vi "WriteCAlexFile.vi"(6 "Overwrite?(F)":bool, 8 "error in (no error)":errorcluster, 10 "Output Path":path, 11 "CAlexData":refnum<class "CAlexData2.lvclass">) -> (0 "error out":errorcluster, 1 "Actual File Name":string, 2 "Output Path dup":path, 3 "CAlexData 2":refnum<class "CAlexData2.lvclass">)   [LabVIEW 2015, in "CAlexData2.lvclass"]
uses:
  CAlexData2.lvclass
  CAlexData2.lvclass/CAlexData2.ctl
  ExpData/ExpData.lvclass
  CustomVIs/CustomVI.lvlib
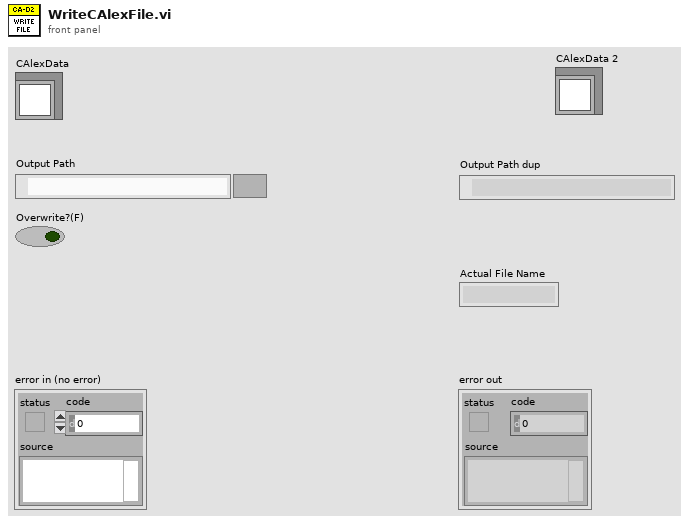
[diagram p1: front panel]
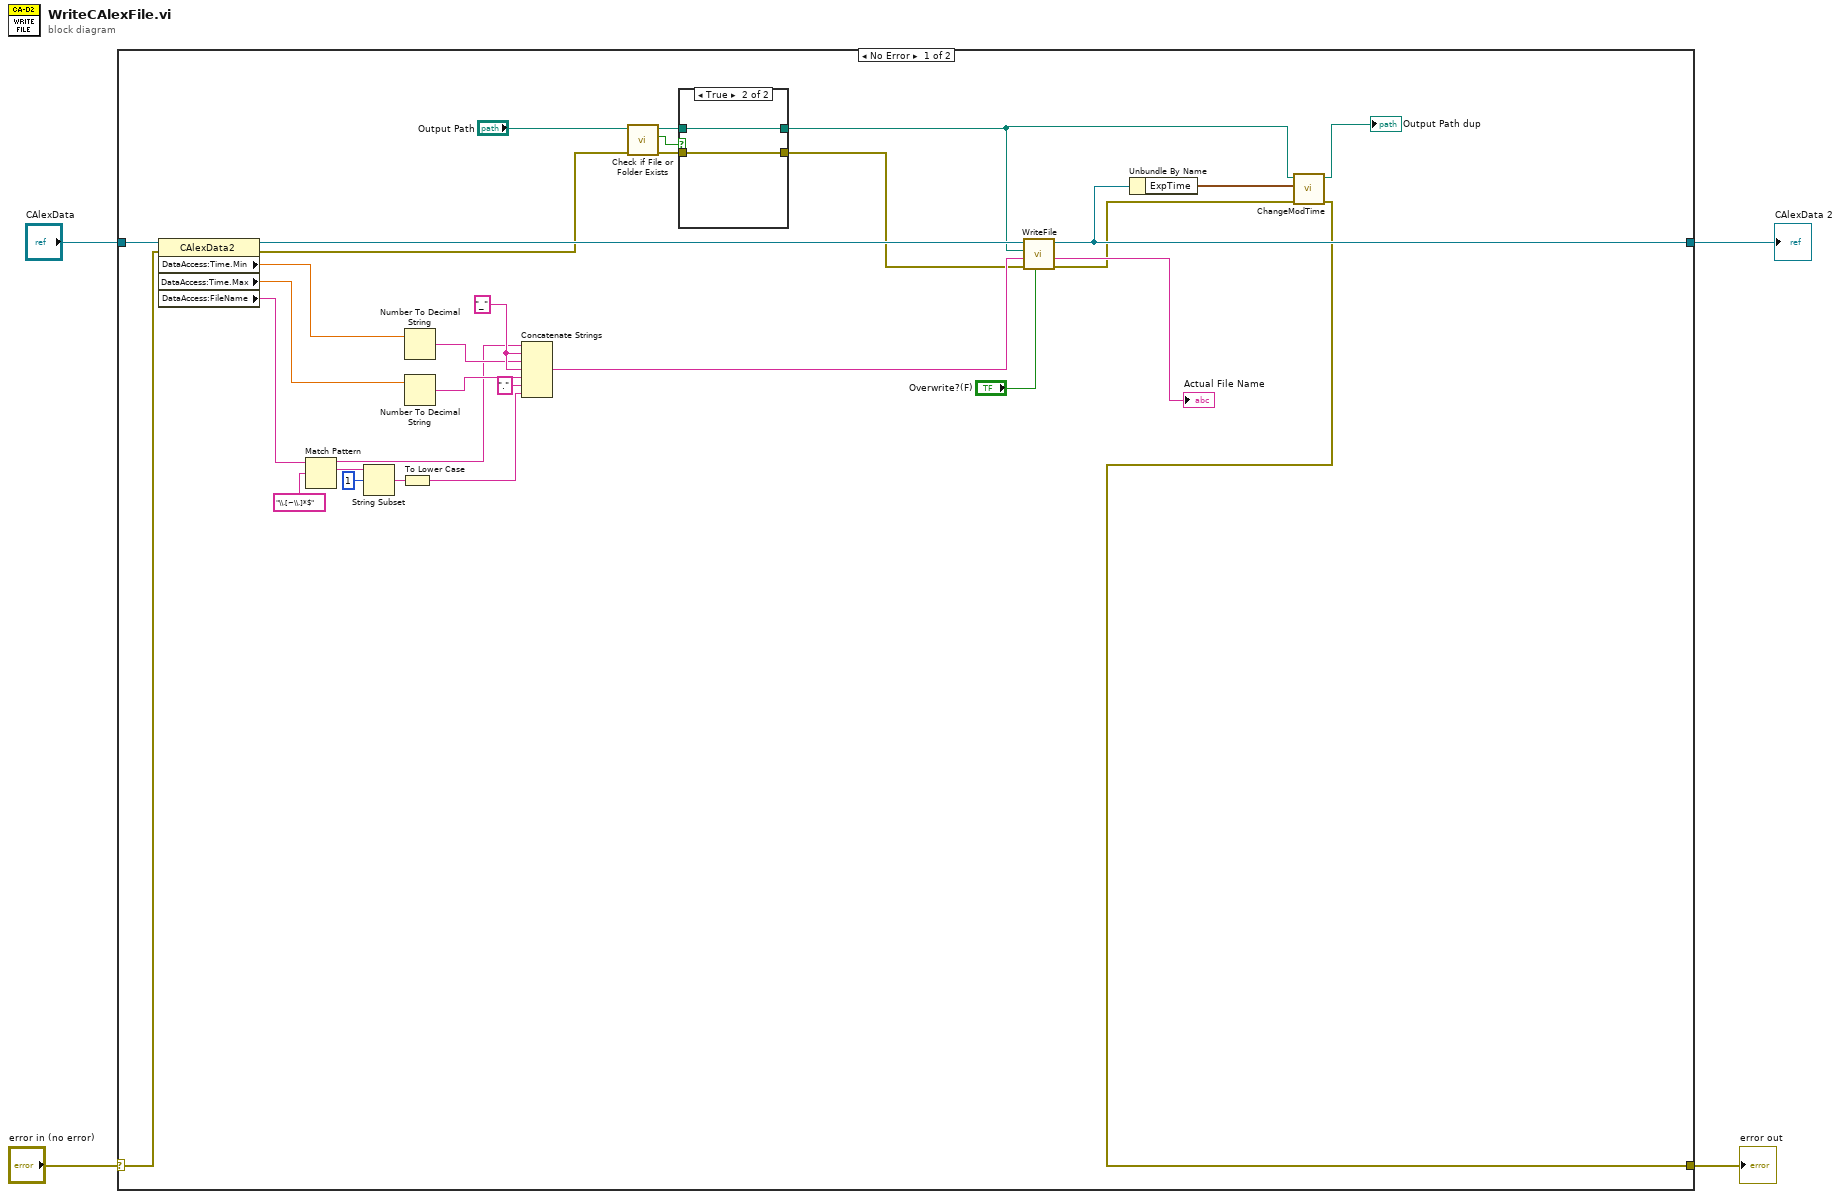
[diagram p0: block diagram]
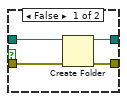
[diagram p2: hidden frame]
diagram:
  n1 = case shown="No Error" "error in (no error)" {
    selector: "error in (no error)" -> [w31 w43]
    tunnel: [w5 w43] -> w3
    tunnel: [w8 w42] -> w1
    tunnel: "CAlexData" -> [w33 w42]
    frame No Error {
      w28 = "_" ("string")
      n2 = property class="CAlexData2"(reference=w33, error in=w31) -> (reference out=w32:refnum<class "CAlexData2.lvclass">, error out=w20:errorcluster, "DataAccess:Time.Min"=w30:dbl, "DataAccess:Time.Max"=w29:dbl, "DataAccess:FileName"=w14:string)
      n3 = Match Pattern(string=w14, regular expression="\\.[~\\.]*$") -> (before substring=w13:string, match substring=w18:string)  [unwired: 3 out]
      n4 = String Subset(string=w18, offset (0)=1) -> (substring=w17:string)  [unwired: 1 out]
      n5 = To Lower Case(string=w17) -> (all lower case string=w11:string)
      n6 = Number To Decimal String(number=w30) -> (decimal integer string=w27:string)  [unwired: 1 in]
      n7 = Number To Decimal String(number=w29) -> (decimal integer string=w26:string)  [unwired: 1 in]
      n8 = Concatenate Strings(w13, w28, w27, w28, w26, "." ("string"), w11) -> (w25:string)
      n9 = call <vilib>:"Check if File or Folder Exists.vi"("error in (no error)"=w20, "path"="Output Path") -> ("error out"=w23:errorcluster, "file or folder exists?"=w24:bool, "dup path"=w22:path)  [unwired: 7 in]
      n10 = case shown="True" w24 {
        tunnel: [w39 w41] -> w10
        tunnel: [w38 w40] -> w21
        tunnel: w22 -> [w37 w41]
        tunnel: w23 -> [w36 w40]
        frame False {
          n11 = Create Folder(path (use dialog)=w37, error in=w36) -> (created path=w39:path, error out=w38:errorcluster)  [unwired: 1 in, 1 out]
        }
        frame True {
        }
      }
      n12 = call "WriteFile.vi"("Overwrite?(F)"="Overwrite?(F)", "error in (no error)"=w21, "Proposed File Name"=w25, "Output Path"=w10, "CarexData In"=w32) -> ("error out"=w6:errorcluster, "Actual File Name"=→"Actual File Name":string, "CarexData Out"=w8:refnum<class "CAlexData2.lvclass">)  [unwired: 4 in]
      n13 = Unbundle By Name(w8) -> ("ExpTime"=w7:timestamp)
      n14 = call "ChangeModTime.vi"("error in (no error)"=w6, "Time Stamp"=w7, "path"=w10) -> ("error out"=w5:errorcluster, "path dup"=→"Output Path dup":path)  [unwired: 7 in]
    }
    frame Error {
    }
  }
  "error out" <- w3
  "CAlexData 2" <- w1
